vi "Configre DPLL.vi"(7 "dpll.channel 0":i32, 8 "error in (no error)":errorcluster, 9 "dpll.q 0":dbl, 10 "dpll.m 0":i8, 11 "LIA Host Interface in":refnum<class "LIA Debugging.lvclass">) -> (0 "error out":errorcluster, 3 "LIA Host Interface Out":refnum<class "LIA Debugging.lvclass">)   [LabVIEW 2017, in "LIA Debugging.lvclass"]
uses:
  LIA Debugging.lvclass
  Shared/lib/interface/Interface FPGA/LIA Host Interface FPGA.lvclass
  Shared/lib/interface/Interface FPGA/Properties/FpgaSession_GET.vi
  <vilib>/Utility/error.llb/Error Cluster From Error Code.vi
  <vilib>/rvi/errors/niLvFpgaAdjustHostInterfaceError.vi
  <vilib>/rvi/interface/nirviReadWriteControl/nirviReadWriteControl.xnode
  <vilib>/rvi/interface/Simulation/niFpgaSimulationCallBeginRW.vi
  NiFpgaLv.dll
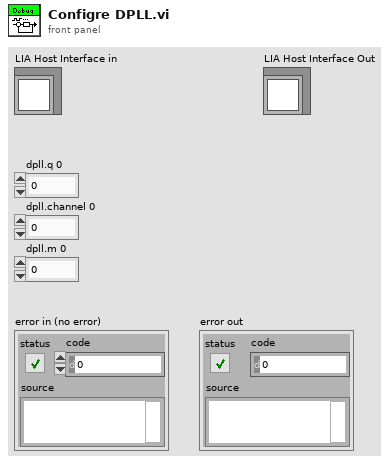
[diagram p1: front panel]
types:
  T1 = cluster{"highLevel":fxp<+/-,18,1>, "lowLevel":fxp<+/-,18,1>, "trigger slope":enum8{"Positive", "Negative"}}
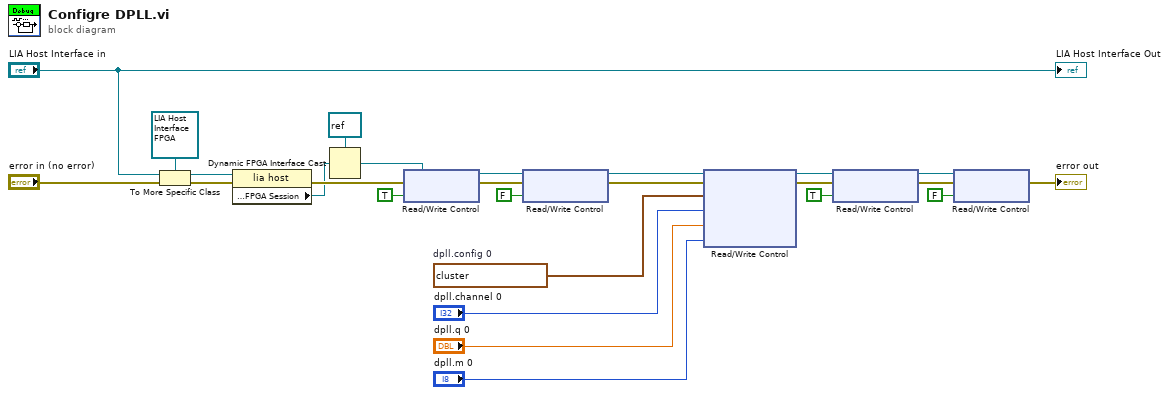
[diagram p0: block diagram]
diagram:
  w17 = T1 {"highLevel"=0.25, "lowLevel"=0.0, "trigger slope"=enum."Positive"}  # dpll.config 0
  n1 = To More Specific Class(target class=refnum<class "LIA Host Interface FPGA.lvclass"> refnum ("lia host"), reference="LIA Host Interface in", error in="error in (no error)") -> (specific class reference=w14:refnum<class "LIA Host Interface FPGA.lvclass">, error out=w13:errorcluster)
  n2 = property class="lia host"(reference=w14, error in=w13) -> (error out=w25:errorcluster, "Properties:FPGA Session"=w15:refnum<k20>)  [unwired: 1 out]
  n3 = Dynamic FPGA Interface Cast(Session In=refnum<k20> refnum ("fpga type"), Type=w15) -> (Session Out=w24:refnum<k20>)
  n4 = xnode "Read/Write Control"("FPGA VI Reference In"=w24, "error in"=w25, "dpll.reset 0"=TRUE) -> ("FPGA VI Reference Out"=w8:refnum<k20>, "error out"=w6:errorcluster)
  n5 = xnode "Read/Write Control"("FPGA VI Reference In"=w8, "error in"=w6, "dpll.enable 0"=FALSE) -> ("FPGA VI Reference Out"=w7:refnum<k20>, "error out"=w5:errorcluster)
  n6 = xnode "Read/Write Control"("FPGA VI Reference In"=w7, "error in"=w5, "dpll.config 0"=w17, "dpll.channel 0"="dpll.channel 0", "dpll.q 0"="dpll.q 0", "dpll.m 0"="dpll.m 0") -> ("FPGA VI Reference Out"=w20:refnum<k20>, "error out"=w21:errorcluster)
  n7 = xnode "Read/Write Control"("FPGA VI Reference In"=w20, "error in"=w21, "dpll.enable 0"=TRUE) -> ("FPGA VI Reference Out"=w3:refnum<k20>, "error out"=w2:errorcluster)
  n8 = xnode "Read/Write Control"("FPGA VI Reference In"=w3, "error in"=w2, "dpll.reset 0"=FALSE) -> ("error out"=→"error out":errorcluster)  [unwired: 1 out]
  "LIA Host Interface Out" <- "LIA Host Interface in"
